vi "CorCheck.vi"(11 "Cohort in":refnum<class "Cohort.lvclass">) -> (0 "error out":errorcluster)   [LabVIEW 2012, in "Cohort.lvclass"]
uses:
  Cohort.lvclass
panel:
  in  "error in (no error)":errorcluster
  in  "Cohort out":refnum<class "Cohort.lvclass">
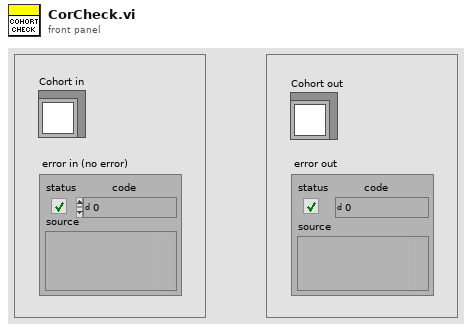
[diagram p1: front panel]
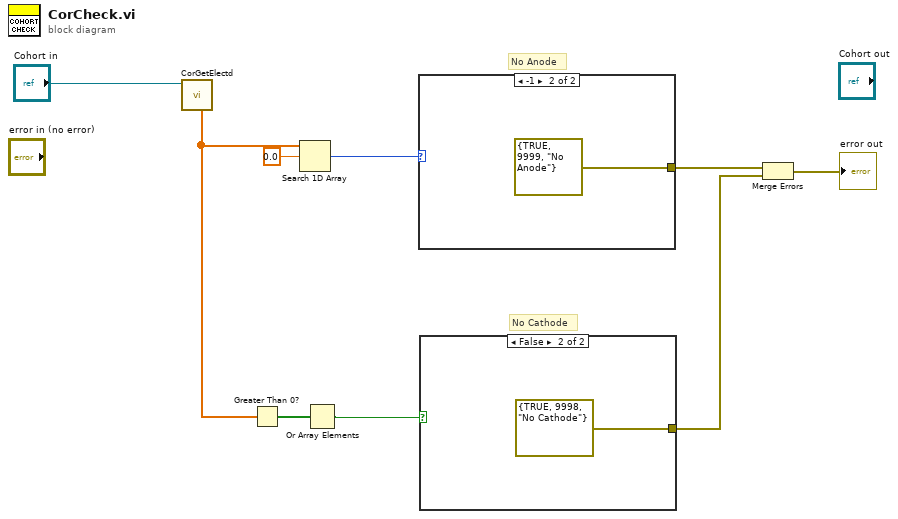
[diagram p0: block diagram]
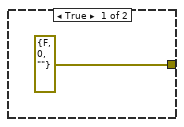
[diagram p2: hidden frame]
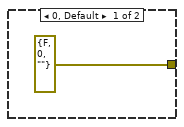
[diagram p3: hidden frame]
diagram:
  # "No Cathode"
  # "No Anode"
  n1 = call-dynamic "CorGetElectd.vi"("Cohort in"="Cohort in") -> ("Amplitude"=w3:sgl[])  [unwired: 6 in, 4 out]
  n2 = Greater Than 0?(x=w3) -> (x > 0?=w2:bool[])
  n3 = Search 1D Array(1D array=w3, element=sgl 0.0) -> (index of element=w7:i32)  [unwired: 1 in]
  n4 = Or Array Elements(Boolean array=w2) -> (logical OR=w1:bool)
  n5 = case shown="-1" w7 {
    tunnel: [errorcluster {"status"=FALSE, "code"=0, "source"=""} ("error constant") errorcluster {TRUE, 9999, "No Anode"}] -> w6
    frame 0, Default {
    }
    frame -1 {
    }
  }
  n6 = case shown="False" w1 {
    tunnel: [errorcluster {"status"=FALSE, "code"=0, "source"=""} ("error constant") errorcluster {TRUE, 9998, "No Cathode"}] -> w5
    frame True {
    }
    frame False {
    }
  }
  n7 = Merge Errors(w6, w5) -> (→"error out":errorcluster)
